vi "Lake Shore 372 Configure Output and Acquire Reading.vi"() -> ()   [LabVIEW 2015]
doc: "This example was designed to demonstrate typical usage of Model 372 sub vi's containing the more common output parameter functions.\n\nThis example configures the control parameters and setpoint of the instrument, allows for a delay, and then reads sensor and heater output data. The user is given the option of just reading data and not configuring the instrument."
uses:
  <instrlib>/Lake Shore 372/Lake Shore 372.lvlib
panel:
  in  "Setpoint Change Delay (25sec)":i32=25 min=1 max=255 step=1
  in  "Filtered Readings (0: Unfiltered)":u16(ring) items=["Unfiltered", "Filtered"]
  in  "Polarity (0: Unipolar)":u16(ring) items=["Unipolar", "Bipolar"]
  in  "Enable Power-up (F: Disable)":bool
  in  "Channel (1:1)":u16(ring)=1 items=["1"=1, "2"=2, "3"=3, "4"=4, "5"=5, "6"=6, "7"=7, "8"=8, "9"=9, "10"=10, "11"=11, "12"=12, "13"=13, "14"=14, "15"=15, "16"=16, "A (Control Input)"=17]
  in  "Output Mode (0: Off)":u16(ring) items=["Off", "Monitor Out", "Open Loop (Manual)", "Zone", "Still", "Closed Loop (PID)", "Warm-up"]
  in  "Warmup % (50%)":dbl=50.0 min=0.0 max=100.0 step=1.0
  in  "Warmup Control (0: Auto off)":u16(ring) items=["Auto off", "Continuous"]
  in  "Rate(D) (0)":dbl min=0.0 max=2500.0 step=1.0 format="%.6f"
  in  "Reset(I) (20)":dbl=20.0 min=0.0 max=10000.0 step=1.0 format="%.6f"
  in  "Gain(P) (10.000)":dbl=10.0 min=0.001 max=1000.0 step=0.001 format="%.6f"
  in  "Heater Range (0: Off)":u16(ring) items=["Off", "31.6 uA", "100 uA", "316 uA", "1.00 mA", "3.16 mA", "10.0 mA", "31.6 mA", "100 mA"]
  in  "Manual Output (0.000%)":dbl min=-100.0 max=100.0 step=0.001 format="%.3f"
  in  "Setpoint (0.00000E+0)":dbl min=0.0 max=100000000.0 step=1e-06 format="%^.5e"
  in  "Output (0: sample heater)":u16(ring) items=["sample heater", "output 1 (warm-up heater) ", "output 2 (analog/still)"]
  out "Quadrature Reading":dbl min=0.0 max=63200000.0 step=1e-05 format="%^.5e"
  out "Heater Output":dbl(slide) min=0.0 max=100.0 step=1e-05 scale=0.0..100.0 scale format="%.2f"
  out "Power Reading":dbl min=0.0 max=0.01 step=1e-05 format="%^.5e"
  out "Kelvin Reading":dbl min=0.0 max=1000.0 step=1e-05 format="%^.5e"
  out "Resistance Reading":dbl min=0.0 max=63200000.0 step=1e-05 format="%^.5e"
  in  "Baud Rate (3: 57600)":i32(ring)=3 items=["300", "1200", "9600", "57600 (USB Only)"]
  in  "VISA resource name":refnum<visa-resource-name>
  in  "Configure (False)":bool
  # "(c) 2015 Advint LLC.  ALL RIGHTS RESERVED."
  # "Control Mode Settings"
  # "Closed Loop Control Settings"
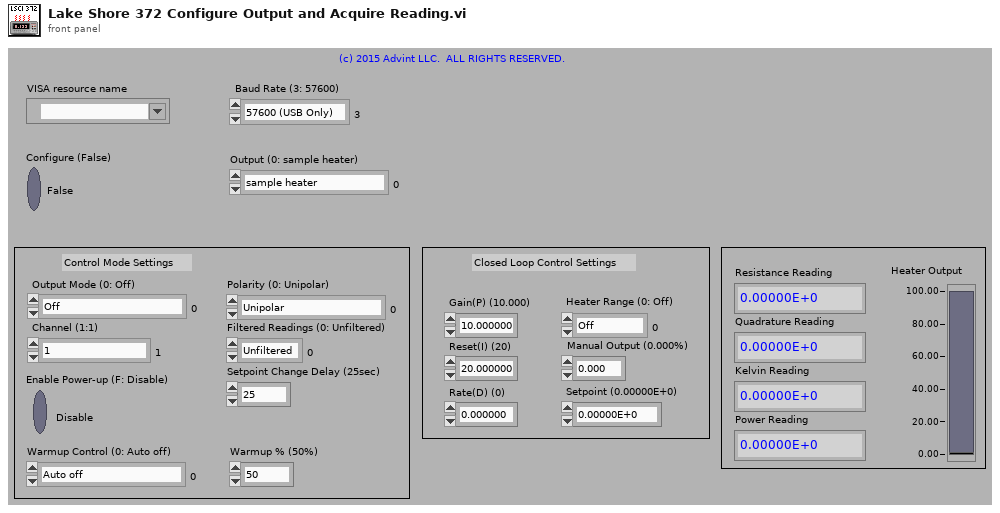
[diagram p1: front panel]
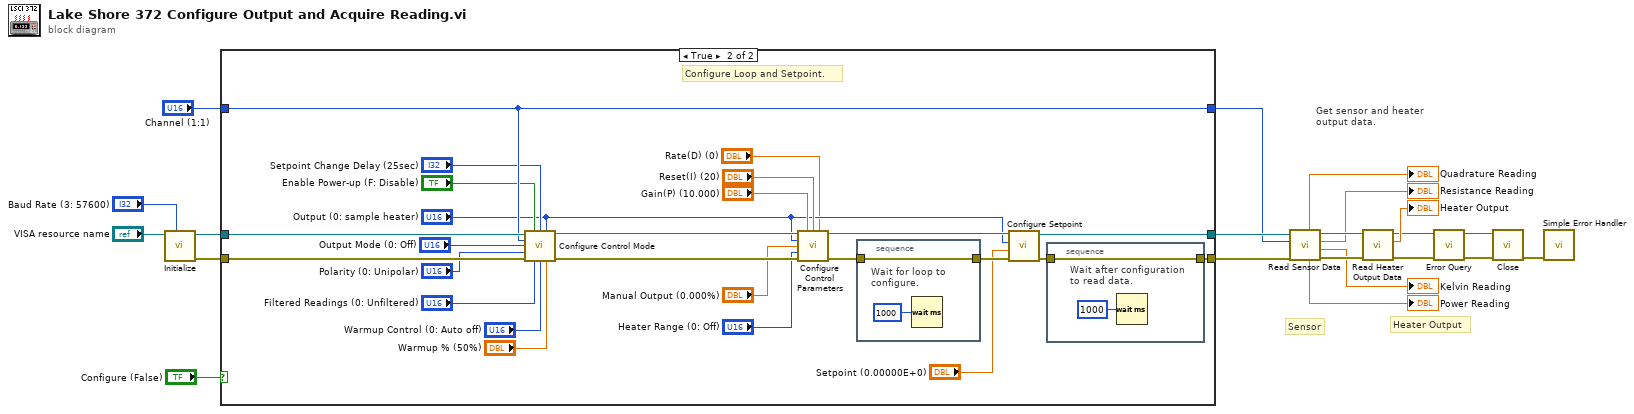
[diagram p0: block diagram]
diagram:
  # "Heater Output"
  # "Sensor"
  # "Get sensor and heater\noutput data."
  n1 = call <instrlib>:"Initialize.vi"("Baud Rate (3: 57600)"="Baud Rate (3: 57600)", "VISA resource name"="VISA resource name") -> ("error out"=w20:errorcluster, "VISA resource name out"=w19:refnum<visa-resource-name>)  [unwired: 8 in]
  n2 = case shown="True" "Configure (False)" {
    tunnel: w20 -> [w23 w39]
    tunnel: w19 -> [w24 w42]
    tunnel: [w23 w49] -> w16
    tunnel: [w24 w44] -> w17
    tunnel: "Channel (1:1)" -> [w22 w34]
    tunnel: [w22 w34] -> w1
    frame False {
      # "Do not configure Loop and Setpoint."
    }
    frame True {
      # "Configure Loop and Setpoint."
      n3 = call <instrlib>:"Configure Control Mode.vi"("VISA resource name"=w42, "Enable Power-up (F: Disable)"="Enable Power-up (F: Disable)", "Setpoint Change Delay (25sec)"="Setpoint Change Delay (25sec)", "Output (0: sample heater)"="Output (0: sample heater)", "Channel (1:1)"=w34, "Output Mode (0: Off)"="Output Mode (0: Off)", "Polarity (0: Unipolar)"="Polarity (0: Unipolar)", "error in (no error)"=w39, "Filtered Readings (0: Unfiltered)"="Filtered Readings (0: Unfiltered)", "Warmup Control (0: Auto off)"="Warmup Control (0: Auto off)", "Warmup % (50%)"="Warmup % (50%)") -> ("VISA resource name out"=w41:refnum<visa-resource-name>, "error out"=w40:errorcluster)  [unwired: 3 in]
      n4 = call <instrlib>:"Configure Control Parameters.vi"("VISA resource name"=w41, "Gain(P) (10.000)"="Gain(P) (10.000)", "Reset(I) (20)"="Reset(I) (20)", "Rate(D) (0)"="Rate(D) (0)", "Output (0: sample heater)"="Output (0: sample heater)", "Manual Output (0.000%)"="Manual Output (0.000%)", "Heater Range (0: Off)"="Heater Range (0: Off)", "error in (no error)"=w40) -> ("VISA resource name out"=w45:refnum<visa-resource-name>, "error out"=w48:errorcluster)  [unwired: 6 in]
      n5 = stacked-sequence {
        tunnel: w48 -> [w52]
        tunnel: [w52] -> w47
        frame #0 {
          # "Wait for loop to \nconfigure."
          n6 = Wait (ms)(milliseconds to wait=u32 1000) -> ()  [unwired: 1 out]
        }
      }
      n7 = call <instrlib>:"Configure Setpoint.vi"("error in (no error)"=w47, "Setpoint (0.00000E+0)"="Setpoint (0.00000E+0)", "Output (0: Sample Heater)"="Output (0: sample heater)", "VISA resource name"=w45) -> ("error out"=w46:errorcluster, "VISA resource name out"=w44:refnum<visa-resource-name>)  [unwired: 6 in]
      n8 = stacked-sequence {
        tunnel: w46 -> [w51]
        tunnel: [w51] -> w49
        frame #0 {
          # "Wait after configuration\nto read data."
          n9 = Wait (ms)(milliseconds to wait=u32 1000) -> ()  [unwired: 1 out]
        }
      }
    }
  }
  n10 = call <instrlib>:"Read Sensor Data.vi"("error in (no error)"=w16, "Channel (1:1)"=w1, "VISA resource name"=w17) -> ("error out"=w15:errorcluster, "Kelvin Reading"=→"Kelvin Reading":dbl, "Resistance Reading"=→"Resistance Reading":dbl, "VISA resource name out"=w14:refnum<visa-resource-name>, "Power Reading"=→"Power Reading":dbl, "Quadrature Reading"=→"Quadrature Reading":dbl)  [unwired: 3 in]
  n11 = call <instrlib>:"Read Heater Output Data.vi"("error in (no error)"=w15, "VISA resource name"=w14) -> ("error out"=w6:errorcluster, "Heater Output"=→"Heater Output":dbl, "VISA resource name out"=w5:refnum<visa-resource-name>)  [unwired: 7 in]
  n12 = call <instrlib>:"Error Query.vi"("error in (no error)"=w6, "VISA resource name"=w5) -> ("error out"=w4:errorcluster, "VISA resource name out"=w3:refnum<visa-resource-name>)  [unwired: 7 in, 1 out]
  n13 = call <instrlib>:"Close.vi"("error in (no error)"=w4, "VISA resource name"=w3) -> ("error out"=w10:errorcluster)  [unwired: 9 in]
  n14 = call <vilib>:"Simple Error Handler.vi"("error in (no error)"=w10) -> ()  [unwired: 4 in, 5 out]
